vi "Relu 3D.vi"(11 "Data In":dbl[][][](array[numeric])) -> (3 "Data out":dbl[][][](array[numeric]))   [LabVIEW 2015]
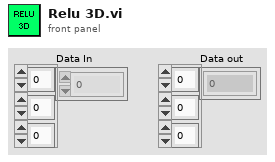
[diagram p1: front panel]
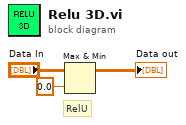
[diagram p0: block diagram]
diagram:
  # "RelU"
  n1 = Max & Min(x="Data In", y=0.0) -> (max(x,y)=→"Data out":dbl[][][])  [unwired: 1 out]
